vi "GE 5565PIORC.VISA.Move In-Place.DBL.vi"(5 "count (-1: all)":i32=-1, 6 "byte order (big-endian)":T1(ring), 7 "address space":T2=1 items=["VXI/VME A16"=1, "VXI/VME A24"=2, "VXI/VME A32"=3, "VXI/VME A64"=4, "PXI Memory Allocations"=9, "PXI Configuration"=10, "PXI BAR0"=11, "PXI BAR1"=12, "PXI BAR2"=13, "PXI BAR3"=14, "PXI BAR4"=15, "PXI BAR5"=16], 8 "error in (no error)":errorcluster, 9 "data in":dbl[](array[numeric]), 10 "offset":u32, 11 "GE 5565PIORC in":refnum<class "GE 5565PIORC.lvclass">) -> (0 "error out":errorcluster, 1 "data out":dbl[](array[numeric]), 3 "GE 5565PIORC out":refnum<class "GE 5565PIORC.lvclass">)   [LabVIEW 2020, in "GE 5565PIORC.lvclass"]
uses:
  GE 5565PIORC.lvclass
  <vilib>/Instr/_visa.llb/VISA Register Access Address Space.ctl
  GE 5565PIORC.lvclass/GE 5565PIORC.ctl
  GE 5565PIORC.VISA.Return Handler.vi
  <vilib>/Utility/error.llb/Error Cluster From Error Code.vi
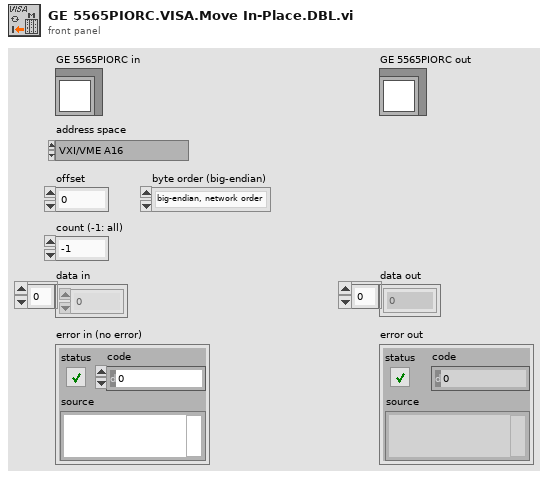
[diagram p1: front panel]
types:
  T1 = enum16{"big-endian, network order", "native, host order", "little-endian"}
  T2 = typedef "VISA Register Access Address Space.ctl" = u16
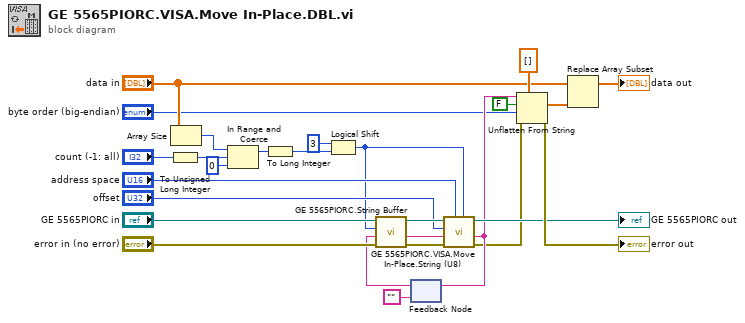
[diagram p0: block diagram]
diagram:
  n1 = To Unsigned Long Integer(number="count (-1: all)") -> (unsigned 32bit integer=w23:u32)
  n2 = Array Size(array="data in") -> (size(s)=w25:i32)
  n3 = In Range and Coerce(upper limit=w25, x=w23, lower limit=u32 0) -> (coerced(x)=w12:u32)  [unwired: 1 out]
  n4 = To Long Integer(number=w12) -> (32bit integer=w2:i32)
  n5 = Logical Shift(y=i16 3, x=w2) -> (x << y=w1:i32)
  n6 = feedback #1("" ("data out")) -> (w15:string)
  n7 = call "GE 5565PIORC.String Buffer.vi"("error in (no error)"="error in (no error)", "string buffer in"=w15, "minimum size"=w1, "GE 5565PIORC in"="GE 5565PIORC in") -> ("error out"=w18:errorcluster, "string buffer out"=w14:string, "GE 5565PIORC out"=w19:refnum<class "GE 5565PIORC.lvclass">)  [unwired: 5 in]
  n8 = call "GE 5565PIORC.VISA.Move In-Place.String (U8).vi"("count (-1: all)"=w1, "address space"="address space", "error in (no error)"=w18, "data in"=w14, "offset"="offset", "GE 5565PIORC in"=w19) -> ("error out"=w3:errorcluster, "data out"=w11:string, "GE 5565PIORC out"=→"GE 5565PIORC out":refnum<class "GE 5565PIORC.lvclass">)  [unwired: 3 in]
  n9 = feedback-in #1(w11) -> ()
  n10 = Unflatten From String(type=dbl[] [], binary string=w11, data includes array or string size? (T)=FALSE, byte order (0:big-endian, network order)="byte order (big-endian)", error in (no error)=w3) -> (value=w8:dbl[], error out=→"error out":errorcluster)  [unwired: 1 out]
  n11 = Replace Array Subset(array="data in", new element=w8) -> (→"data out":dbl[])  [unwired: 1 in]
